vi "flash_vna_generator.vi"(2 "error in":errorcluster) -> (0 "error out":errorcluster)   [LabVIEW 2013]
doc: "Runs before the main program, to ensure that VNA is switched on and the temperature log file is loaded"
panel:
  in  "Boolean 3":bool=TRUE
  in  "Boolean 2":bool
  in  "Boolean":bool
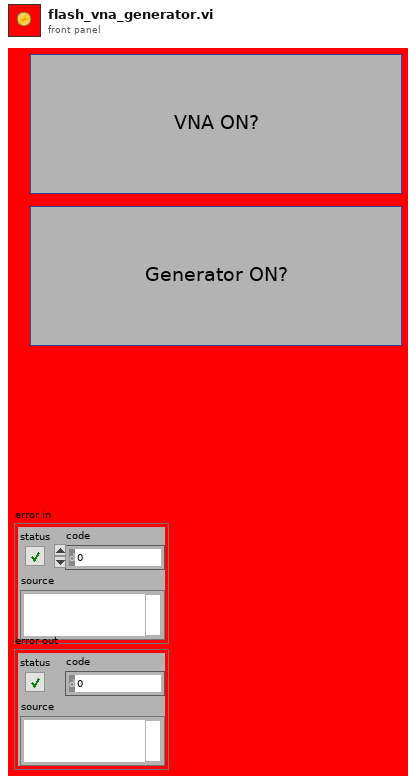
[diagram p1: front panel]
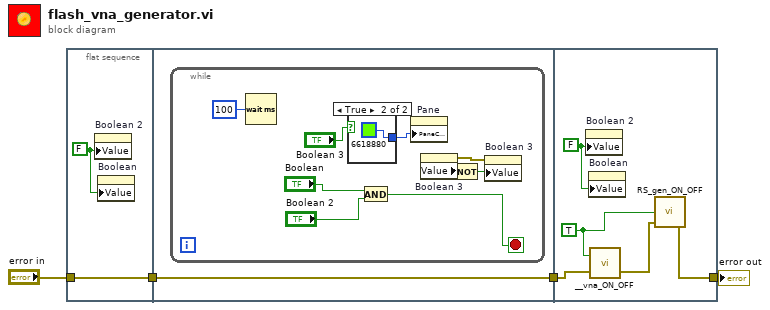
[diagram p0: block diagram]
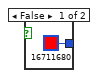
[diagram p2: hidden frame]
diagram:
  n1 = flat-sequence {
    tunnel: "error in" -> [w6]
    tunnel: [w6] -> w1
    tunnel: [w7] -> w3
    tunnel: w1 -> [w7]
    tunnel: [w21] -> w2
    tunnel: w3 -> [w22]
    frame #0 {
      w5 = FALSE ("Boolean 2")
      n2 = property on="Boolean 2" class="Bool (strict)"("Value"=w5) -> ()  [unwired: 2 in, 2 out]
      n3 = property on="Boolean" class="Bool (strict)"("Value"=w5) -> ()  [unwired: 2 in, 2 out]
    }
    frame #1 {
      n4 = while {
        stop <- w14 stop-if-true
        n5 = Wait (ms)(milliseconds to wait=u32 100) -> ()  [unwired: 1 out]
        n6 = case shown="True" "Boolean 3" {
          tunnel: [u32 16711680 u32 6618880] -> w13
          frame False {
          }
          frame True {
          }
        }
        n7 = And(x="Boolean", y="Boolean 2") -> (x .and. y?=w14:bool)
        n8 = property on="Pane" class="Pane"("PaneColor"=w13) -> ()  [unwired: 2 in, 2 out]
        n9 = property on="Boolean 3" class="Bool (strict)"() -> (error out=w12:errorcluster, "Value"=w11:bool)  [unwired: 2 in, 1 out]
        n10 = Not(x=w11) -> (.not. x?=w10:bool)
        n11 = property on="Boolean 3" class="Bool (strict)"(error in=w12, "Value"=w10) -> ()  [unwired: 1 in, 2 out]
      }
    }
    frame #2 {
      w19 = TRUE ("Boolean 2")
      w23 = FALSE ("Boolean 2")
      n12 = property on="Boolean 2" class="Bool (strict)"("Value"=w23) -> ()  [unwired: 2 in, 2 out]
      n13 = property on="Boolean" class="Bool (strict)"("Value"=w23) -> ()  [unwired: 2 in, 2 out]
      n14 = call "__vna_ON_OFF.vi"("VNA Output"=w19, "error in (no error)"=w22) -> ("error out"=w20:errorcluster)
      n15 = call "RS_gen_ON_OFF.vi"("error in"=w20, "Generator Output"=w19) -> ("error out"=w21:errorcluster)  [unwired: 3 in]
    }
  }
  "error out" <- w2
